vi "AIN.vi"(0 "VISA resource name":refnum<visa-resource-name>, 1 "error in (no error)":errorcluster) -> (2 "VISA resource Salida":refnum<visa-resource-name>, 3 "AIN data":i16, 4 "error out":errorcluster)   [LabVIEW 2011]
panel:
  out "unsigned byte array":u8[](array[numeric])
  out "Sent":u32
  out "Received":u32
  out "subarray":u8[](array[numeric])
  out "Read AIN command":u8[](array[numeric])
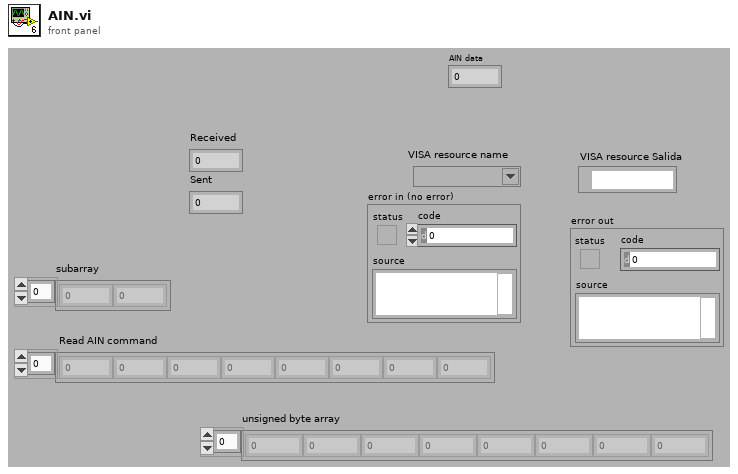
[diagram p1: front panel]
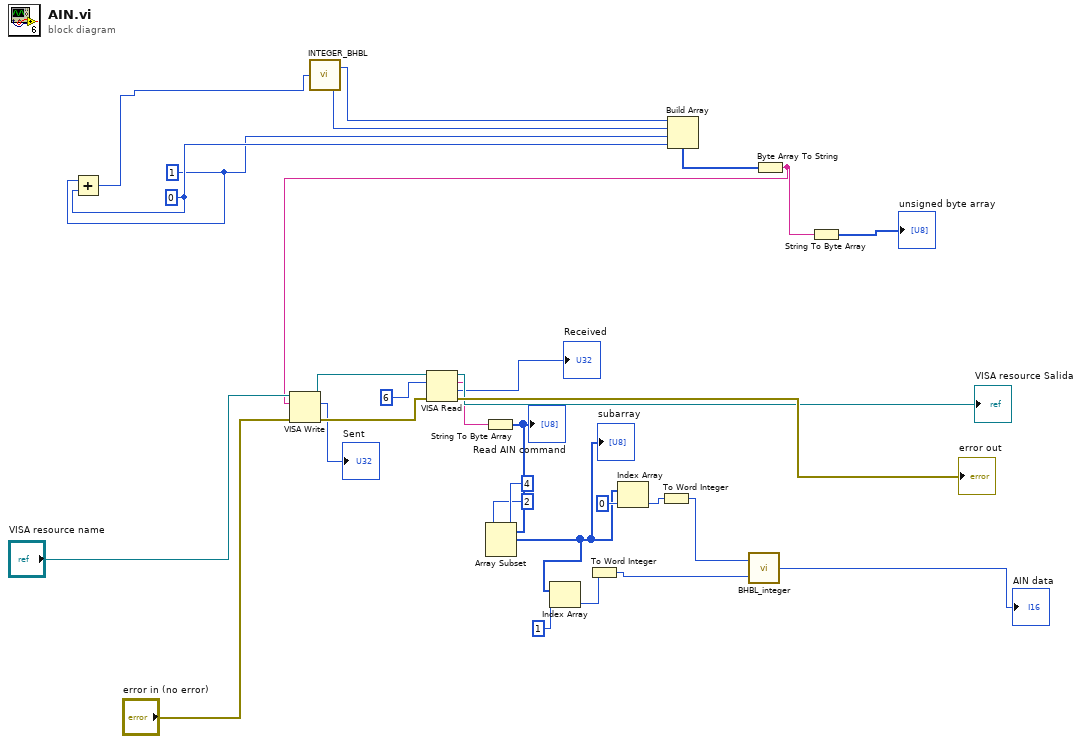
[diagram p0: block diagram]
diagram:
  w7 = i8 1 ("element")
  w8 = i8 0 ("element")
  n1 = Add(x=w7, y=w8) -> (x+y=w4:i8)
  n2 = call "INTEGER_BHBL.vi"("int16"=w4) -> ("Lvalue"=w9:u8, "HValue"=w10:u8)
  n3 = Build Array(w10, w9, w7, w8) -> (w15:u8[])
  n4 = Byte Array To String(unsigned byte array=w15) -> (string=w6:string)
  n5 = VISA Write(VISA resource name="VISA resource name", write buffer=w6, error in (no error)="error in (no error)") -> (VISA resource name out=w26:refnum<visa-resource-name>, return count=→"Sent":u32, error out=w29:errorcluster)
  n6 = VISA Read(VISA resource name=w26, byte count=u32 6, error in (no error)=w29) -> (VISA resource name out=→"VISA resource Salida":refnum<visa-resource-name>, read buffer=w25:string, return count=→"Received":u32, error out=→"error out":errorcluster)
  n7 = String To Byte Array(string=w25) -> (unsigned byte array=w23:u8[])
  "Read AIN command" <- w23
  n8 = Array Subset(array=w23, index=4, length=2) -> (w19:u8[])
  "subarray" <- w19
  n9 = Index Array(array=w19, index=1) -> (element=w16:u8)
  n10 = To Word Integer(number=w16) -> (16bit integer=w2:i16)
  n11 = Index Array(array=w19, index=0) -> (element=w17:u8)
  n12 = To Word Integer(number=w17) -> (16bit integer=w3:i16)
  n13 = call "BHBL_integer.vi"("lo(x)"=w2, "hi(x)"=w3) -> ("(hi.lo)"=→"AIN data":i16)
  n14 = String To Byte Array(string=w6) -> (unsigned byte array=→"unsigned byte array":u8[])
